vi "GUID.vi"() -> (0 "Guid":string)   [LabVIEW 2021, in "Vision.lvlib" / "Vision.lvclass"]
uses:
  Vision.lvclass
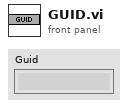
[diagram p1: front panel]
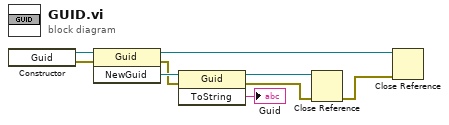
[diagram p0: block diagram]
diagram:
  n1 = constructor class="Guid"() -> (reference out=w9:refnum<k24>, error out=w7:errorcluster)  [unwired: 3 in, 1 out]
  n2 = invoke class="Guid" method="NewGuid"(reference=w9, error in=w7) -> (reference out=w3:refnum<k24>, error out=w6:errorcluster, "NewGuid"=w8:refnum<k24>)  [unwired: 1 in]
  n3 = invoke class="Guid" method="ToString"(reference=w8, error in=w6) -> (reference out=w5:refnum<k24>, error out=w4:errorcluster, "ToString"=→"Guid":string)  [unwired: 1 in]
  n4 = Close Reference(reference=w5, error in (no error)=w4) -> (error out=w2:errorcluster)
  n5 = Close Reference(reference=w3, error in (no error)=w2) -> ()  [unwired: 1 out]
